vi "Translate All UI Strings.vi"(8 "error in (no error)":errorcluster, 9 "Language Index (0)":i32, 10 "Preview?":bool, 11 "LanguageData in":refnum<class "VI Data.lvclass">) -> (0 "error out":errorcluster, 3 "LanguageData out":refnum<class "VI Data.lvclass">)   [LabVIEW 2013, in "SET Project Data.lvlib" / "VI Data.lvclass"]
uses:
  VI Data.lvclass
  VI Data.lvclass/VI Data.ctl
  Control Classes/GObject/GObject.lvclass
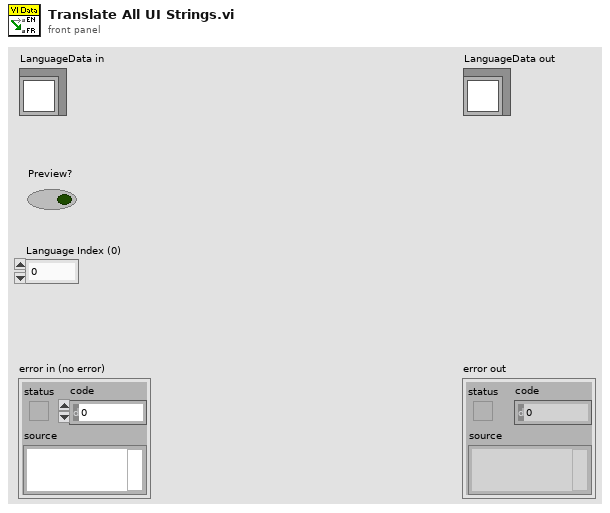
[diagram p1: front panel]
types:
  T1 = enum32{"Invalid", "Standard", "Closed", "Hidden", "Minimized", "Maximized"}
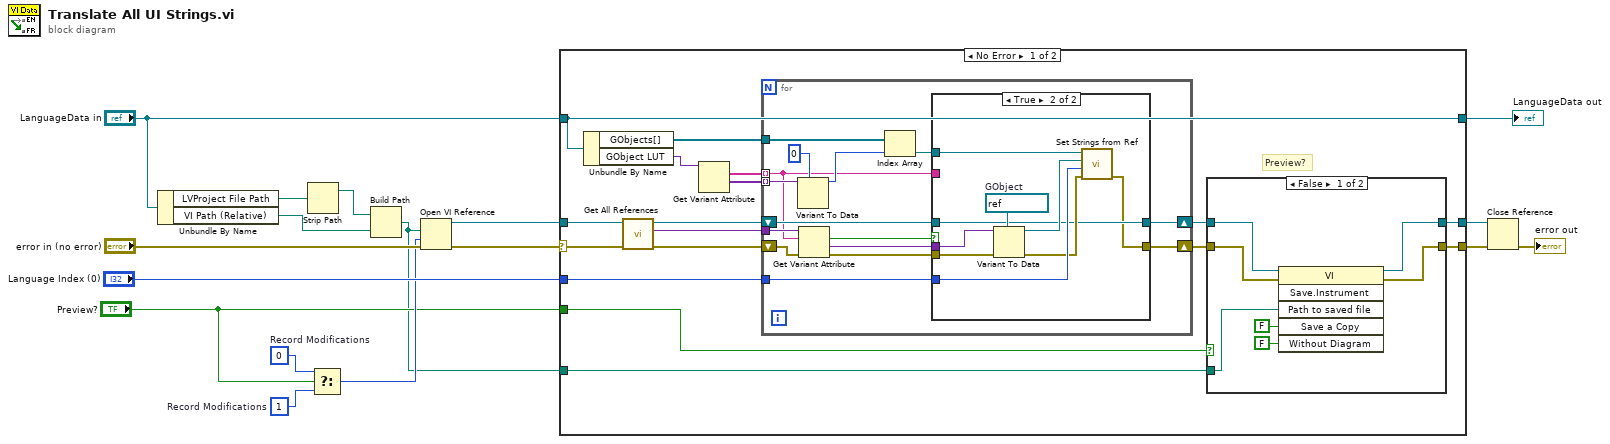
[diagram p0: block diagram]
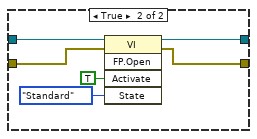
[diagram p2: hidden frame]
diagram:
  w6 = 0  # Record Modifications
  w7 = 1  # Record Modifications
  n1 = Unbundle By Name("LanguageData in") -> ("LVProject File Path"=w10:path, "VI Path (Relative)"=w12:path)
  n2 = Strip Path(path=w10) -> (stripped path=w11:path)  [unwired: 1 out]
  n3 = Select(t=w6, s="Preview?", f=w7) -> (s? t:f=w5:i32)
  n4 = Build Path(base path=w11, name or relative path=w12) -> (appended path=w3:path)
  n5 = Open VI Reference(vi path=w3, options=w5, error in (no error)="error in (no error)") -> (vi reference=w1:refnum<vi>, error out=w2:errorcluster)  [unwired: 3 in]
  n6 = case shown="No Error" w2 {
    selector: w2 -> [w18 w76]
    tunnel: [w25 w76] -> w15
    tunnel: [w29 w75] -> w17
    tunnel: "LanguageData in" -> [w29 w75]
    tunnel: "Language Index (0)" -> [w30 _]
    tunnel: w1 -> [w22 w74]
    tunnel: [w27 w74] -> w14
    tunnel: "Preview?" -> [w24 _]
    tunnel: w3 -> [w23 _]
    frame No Error {
      # "Preview?"
      n7 = Unbundle By Name(w29) -> ("GObjects[]"=w31:refnum<class "GObject.lvclass">[], "GObject LUT"=w34:variant)
      n8 = call "Get All References.vi"("error in (no error)"=w18, "VI Refnum in"=w22) -> ("error out"=w20:errorcluster, "CtlRef LUT"=w19:variant, "VI Refnum out"=w21:refnum<vi>)  [unwired: 7 in]
      n9 = Get Variant Attribute(Variant=w34) -> (names=w33:string[], values=w32:variant[])  [unwired: 3 in, 2 out]
      n10 = for {
        tunnel: w30 -> [w60]
        shift-right: [w58] -> w26
        shift-left: w20 -> [w59]
        tunnel: w31 -> [w62]
        tunnel: w33 -> [w49] mode=indexing
        tunnel: w19 -> [w61]
        tunnel: w32 -> [w57] mode=indexing
        shift-right: [w48] -> w28
        shift-left: w21 -> [w50]
        n11 = Variant To Data(type=0, Variant=w57) -> (data=w52:i32)  [unwired: 1 in, 1 out]
        n12 = Get Variant Attribute(Variant=w61, name=w49, error in=w59) -> (found=w51:bool, value=w56:variant, error out=w55:errorcluster)  [unwired: 1 in, 1 out]
        n13 = Index Array(array=w62, index=w52) -> (element=w54:refnum<class "GObject.lvclass">)
        n14 = case shown="True" w51 {
          tunnel: w56 -> [_ w72]
          tunnel: w60 -> [_ w70]
          tunnel: w55 -> [w64 w69]
          tunnel: [w64 w65] -> w58
          tunnel: w54 -> [_ w67]
          tunnel: w50 -> [w63 w66]
          tunnel: w49 -> [_ _]
          tunnel: [w63 w66] -> w48
          frame False {
          }
          frame True {
            w73 = refnum<vi> refnum  # GObject
            n15 = Variant To Data(error in=w69, type=w73, Variant=w72) -> (data=w71:refnum<vi>, error out=w68:errorcluster)
            n16 = call-dynamic "Set Strings from Ref.vi"("error in (no error)"=w68, "Language Index (0)"=w70, "GObj Refnum"=w71, "GObject in"=w67) -> ("error out"=w65:errorcluster)  [unwired: 6 in, 1 out]
          }
        }
      }
      n17 = case shown="False" w24 {
        tunnel: w28 -> [w38 w47]
        tunnel: [w37 w46] -> w27
        tunnel: w26 -> [w40 w45]
        tunnel: [w39 w44] -> w25
        tunnel: w23 -> [w41 _]
        frame False {
          n18 = invoke class="VI" method="Save.Instrument"(reference=w38, error in=w40, "Path to saved file"=w41, "Save a Copy"=FALSE, "Without Diagram"=FALSE) -> (reference out=w37:refnum<vi>, error out=w39:errorcluster)  [unwired: 1 in, 4 out]
        }
        frame True {
          n19 = invoke class="VI" method="FP.Open"(reference=w47, error in=w45, "Activate"=TRUE ("Activate?"), "State"=T1."Standard") -> (reference out=w46:refnum<vi>, error out=w44:errorcluster)  [unwired: 1 in, 3 out]
        }
      }
    }
    frame Error {
      # "#ERROR - Failed to load VI"
    }
  }
  "LanguageData out" <- w17
  n20 = Close Reference(reference=w14, error in (no error)=w15) -> (error out=→"error out":errorcluster)
